vi "CloseClk.vi"(8 "error in (no error)":errorcluster, 10 "ClkName":string, 11 "NiPxi6683H in":refnum<class "NiPxi6683H.lvclass">) -> (0 "error out":errorcluster, 3 "NiPxi6683H out":refnum<class "NiPxi6683H.lvclass">)   [LabVIEW 2014, in "SyncPlugins.lvlib" / "NiPxi6683H.lvclass"]
uses:
  NiPxi6683H.lvclass
  NiPxi6683H.lvclass/NiPxi6683H.ctl
  NiPxi6682/NiPxi6682.lvclass/NiPxi6682.ctl
  Accessors/Write Clocks.vi
  NiPxi6682/Accessors/Read NiSyncHandle.vi
  Accessors/Read Clocks.vi
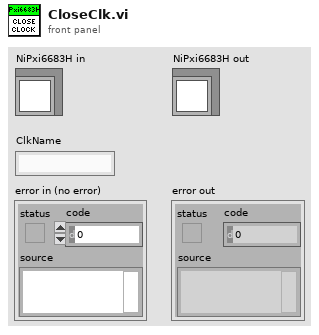
[diagram p1: front panel]
types:
  T1 = typedef "SyncPlugins.lvlib/PXI_MultiTrig.lvclass/clClocks.ctl" = cluster{"Name":string, "RefClk":string, "ClkTerminal":string, "Frequency":dbl, "DutyCycle":dbl, "ClkType":string, "Initiated":bool, "TrigTime":bool}
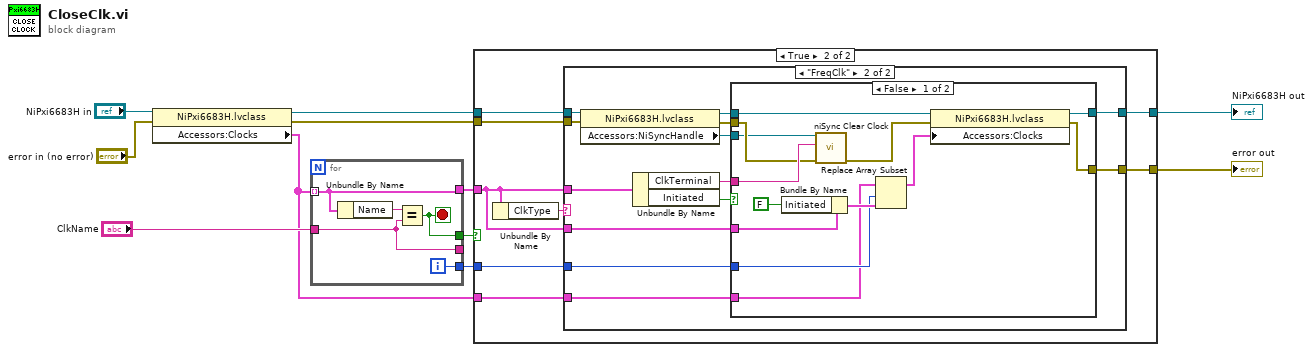
[diagram p0: block diagram]
diagram:
  n1 = property class="NiPxi6683H.lvclass"(reference="NiPxi6683H in", error in="error in (no error)") -> (reference out=w6:refnum<class "NiPxi6683H.lvclass">, error out=w5:errorcluster, "Accessors:Clocks"=w1:T1[])
  n2 = for {
    tunnel: w1 -> [w15] mode=indexing
    tunnel: "ClkName" -> [w13]
    tunnel: [w15] -> w7
    tunnel: [w14] -> w8
    tunnel: [w13] -> _
    tunnel: [w12] -> w2
    i -> [w12]
    stop <- w14 stop-if-true
    n3 = Unbundle By Name(w15) -> ("Name"=w16:string)
    n4 = Equal?(x=w16, y=w13) -> (x = y?=w14:bool)
  }
  n5 = case shown="True" w8 {
    tunnel: w7 -> [_ w21]
    tunnel: w6 -> [w18 w25]
    tunnel: w5 -> [w17 w24]
    tunnel: [w18 w23] -> w4
    tunnel: [w17 w22] -> w3
    tunnel: w2 -> [_ w20]
    tunnel: w1 -> [_ w19]
    frame False {
    }
    frame True {
      n6 = Unbundle By Name(w21) -> ("ClkType"=w26:string)
      n7 = case shown="\"FreqClk\"" w26 {
        tunnel: w25 -> [w28 w41]
        tunnel: w24 -> [w27 w40]
        tunnel: w21 -> [_ w39]
        tunnel: [w28 w33] -> w23
        tunnel: [w27 w29] -> w22
        tunnel: w21 -> [_ w32]
        tunnel: w20 -> [_ w31]
        tunnel: w19 -> [_ w30]
        frame Default {
        }
        frame "FreqClk" {
          n8 = property class="NiPxi6683H.lvclass"(reference=w41, error in=w40) -> (reference out=w35:refnum<class "NiPxi6683H.lvclass">, error out=w34:errorcluster, "Accessors:NiSyncHandle"=w36:refnum<k15>)
          n9 = Unbundle By Name(w39) -> ("ClkTerminal"=w37:string, "Initiated"=w38:bool)
          n10 = case shown="False" w38 {
            tunnel: w37 -> [w54 _]
            tunnel: w36 -> [w49 _]
            tunnel: w35 -> [w51 w56]
            tunnel: w34 -> [w50 w55]
            tunnel: [w45 w56] -> w33
            tunnel: w32 -> [w53 _]
            tunnel: w31 -> [w47 _]
            tunnel: w30 -> [w46 _]
            tunnel: [w42 w55] -> w29
            frame False {
              n11 = Bundle By Name(cluster=w53, "Initiated"=FALSE) -> (w48:T1)
              n12 = call <instrlib>:"niSync Clear Clock.vi"("error in (no error)"=w50, "terminal"=w54, "instrument handle"=w49) -> ("error out"=w43:errorcluster)  [unwired: 6 in, 1 out]
              n13 = Replace Array Subset(array=w46, new element=w48, index=w47) -> (w44:T1[])
              n14 = property class="NiPxi6683H.lvclass"(reference=w51, error in=w43, "Accessors:Clocks"=w44) -> (reference out=w45:refnum<class "NiPxi6683H.lvclass">, error out=w42:errorcluster)
            }
            frame True {
            }
          }
        }
      }
    }
  }
  "error out" <- w3
  "NiPxi6683H out" <- w4
